vi "Untitled 2 (SubVI).vi"(11 "data in":string) -> (3 "data out":string)   [LabVIEW 2018]
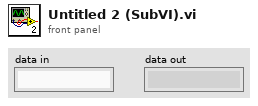
[diagram p1: front panel]
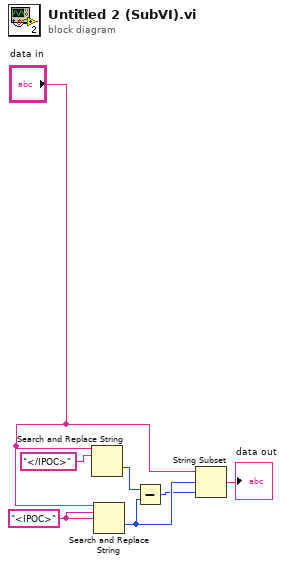
[diagram p0: block diagram]
diagram:
  w4 = "<IPOC>" ("search string")
  n1 = Search and Replace String(input string="data in", search string="</IPOC>") -> (offset past replacement=w3:i32)  [unwired: 6 in, 3 out]
  n2 = Search and Replace String(input string="data in", search string=w4, replace string=w4) -> (offset past replacement=w2:i32)  [unwired: 5 in, 3 out]
  n3 = Subtract(x=w3, y=w2) -> (x-y=w1:i32)
  n4 = String Subset(string="data in", offset (0)=w2, length (rest)=w1) -> (substring=→"data out":string)
